vi "Timeout mS.vi"(10 "Deadline":dbl) -> (2 "Timeout mS":i32)   [LabVIEW 2020, in "OAuth2.lvlib" / "OAuth2.lvclass"]
uses:
  OAuth2.lvclass
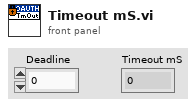
[diagram p1: front panel]
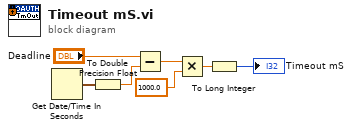
[diagram p0: block diagram]
diagram:
  n1 = Get Date/Time In Seconds() -> (seconds since 1Jan1904=w7:timestamp)
  n2 = To Double Precision Float(number=w7) -> (double precision float=w5:dbl)
  n3 = Subtract(x="Deadline", y=w5) -> (x-y=w4:dbl)
  n4 = Multiply(x=w4, y=1000.0) -> (x*y=w2:dbl)
  n5 = To Long Integer(number=w2) -> (32bit integer=→"Timeout mS":i32)
